vi "C4Dev_waitForEvent.vi"(0 "c4dev in":refnum<k24>, 11 "error in":errorcluster, 12 "timeout_ms in":i64=10000) -> (4 "c4dev out":refnum<k24>, 6 "feature names out":string[](array[string]), 15 "error out":errorcluster)   [LabVIEW 2015, in "libC4HdlLV.lvlib"]
uses:
  libC4HdlLV.lvlib
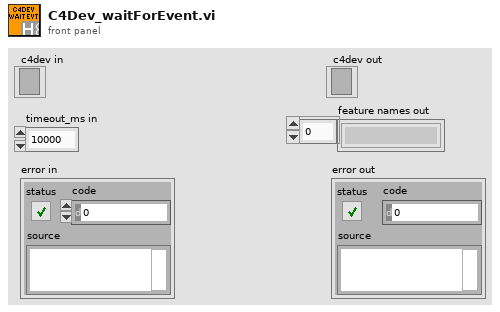
[diagram p1: front panel]
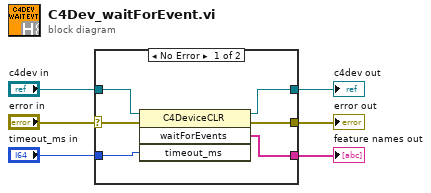
[diagram p0: block diagram]
diagram:
  n1 = case shown="No Error" "error in" {
    selector: "error in" -> [w10 w14]
    tunnel: [w9 w14] -> w5
    tunnel: "c4dev in" -> [w12 w13]
    tunnel: [w11 w13] -> w3
    tunnel: "timeout_ms in" -> [w8 _]
    tunnel: [w7 _] -> w1
    frame No Error {
      n2 = invoke class="C4DeviceCLR" method="waitForEvents"(reference=w12, error in=w10, "timeout_ms"=w8) -> (reference out=w11:refnum<k24>, error out=w9:errorcluster, "waitForEvents"=w7:string[])  [unwired: 1 in, 1 out]
    }
    frame Error {
    }
  }
  "error out" <- w5
  "c4dev out" <- w3
  "feature names out" <- w1
